vi "EnumAndStringbasedCaseStructure.vi"() -> ()   [LabVIEW 2019]
panel:
  in  "States":T1(ring)
  in  "String":string
  in  "Numeric":u8
  in  "Boolean":bool
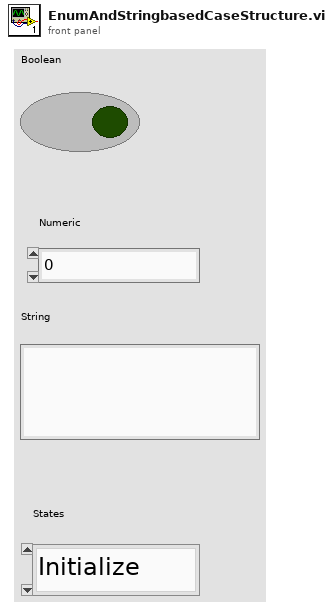
[diagram p1: front panel]
types:
  T1 = enum16{"Initialize", "Process", "Process1", "Exit", "MacroExit"}
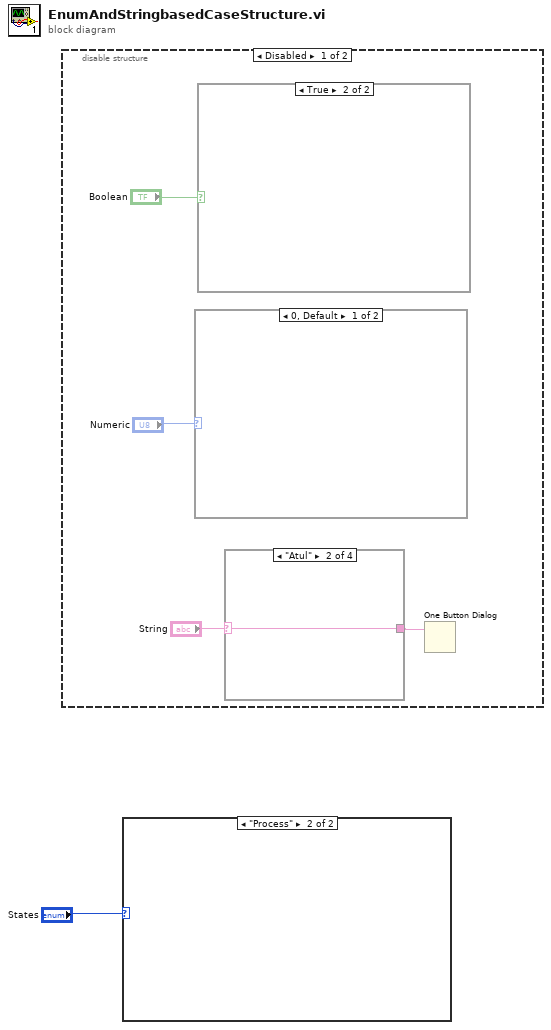
[diagram p0: block diagram]
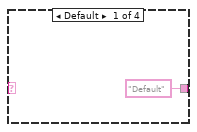
[diagram p3: hidden frame]
diagram:
  n1 = disable-structure shown="Disabled" {
    frame Disabled {
      n2 = case shown="0, Default" "Numeric" {
        frame 0, Default {
        }
        frame 1 {
        }
      }
      n3 = case shown="True" "Boolean" {
        frame False {
        }
        frame True {
        }
      }
      n4 = case shown="\"Atul\"" "String" {
        selector: "String" -> [_ w7 w8 w9]
        tunnel: ["Default" w7 w8 w9] -> w3
        frame Default {
        }
        frame "Atul" {
        }
        frame "Akshay" {
        }
        frame "Joel" {
        }
      }
      n5 = One Button Dialog(message=w3) -> ()  [unwired: 1 in, 1 out]
    }
    frame Enabled {
    }
  }
  n6 = case shown="\"Process\"" "States" {
    frame "Initialize", Default {
    }
    frame "Process" {
    }
  }
